vi "AB_850_860_Project_Source.vi"(7 "action":T4, 8 "error in (no error)":errorcluster, 9 "index in":i32, 10 "dataSource in":T3, 11 "buildObject":T1) -> (0 "error out":errorcluster, 1 "index out":i32, 2 "dataSource out":T3, 3 "buildObject out":T1)   [LabVIEW 2020]
doc: "Reads and writes the data to the object property bag."
uses:
  <resource>/Framework/Providers/API/ItemRef.ctl
  <vilib>/AppBuilder/AB_Source_Inclusion.ctl
  <vilib>/AppBuilder/RW_Project/AB_RW_Project_PropBag_Action.ctl
  <vilib>/AppBuilder/AB_Source_Property_WindowBehavior.ctl
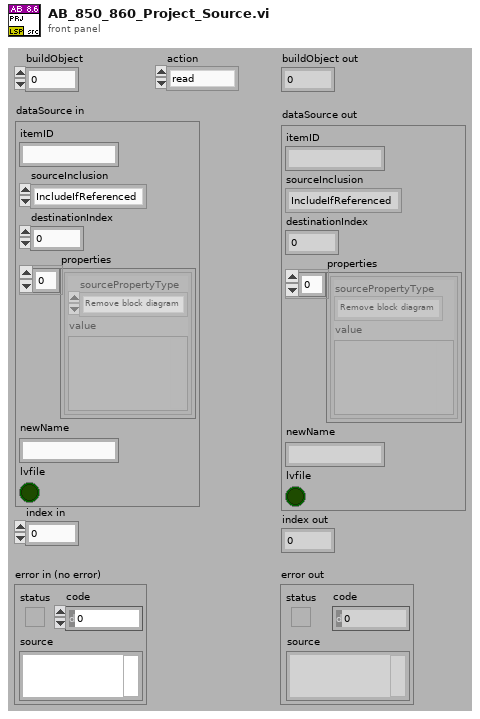
[diagram p1: front panel]
types:
  T1 = typedef "ItemRef.ctl" = u64
  T2 = typedef "AB_Source_Inclusion.ctl" = enum16{"IncludeIfReferenced", "Include", "Exclude", "TopLevel"}
  T3 = cluster{"itemID":string, "sourceInclusion":T2, "destinationIndex":i32, "properties":cluster{"sourcePropertyType":enum16{"Remove block diagram", "Remove front panel", "Password", "Window has title bar", "Show menu bar", "Show vertical scroll bar", "Show horizontal scroll bar", "Show toolbar", "Show Abort button", "Show fp when called", "Window behavior", "Allow user to close window", "Window run-time position", "Run when opened", "Allow debugging", "Auto error handling", "Generate guard code", "Use stack variables", "Expression folding", "Integer only", "Inline subVI"}, "value":variant}[], "newName":string, "lvfile":bool}
  T4 = typedef "AB_RW_Project_PropBag_Action.ctl" = enum16{"read", "write", "clear", "readPrevious", "writePrevious", "clearPrevious"}
  T5 = cluster{"sourcePropertyType":enum16{"Remove block diagram", "Remove front panel", "Password", "Window has title bar", "Show menu bar", "Show vertical scroll bar", "Show horizontal scroll bar", "Show toolbar", "Show Abort button", "Show fp when called", "Window behavior", "Allow user to close window", "Window run-time position", "Run when opened", "Allow debugging", "Auto error handling", "Generate guard code", "Use stack variables", "Expression folding", "Integer only", "Inline subVI"}, "value":variant}
  T6 = typedef "AB_Source_Property_WindowBehavior.ctl" = enum16{"Default", "Floating", "Modal"}
  T7 = enum16{"Remove block diagram", "Remove front panel", "Password", "Window has title bar", "Show menu bar", "Show vertical scroll bar", "Show horizontal scroll bar", "Show toolbar", "Show Abort button", "Show fp when called", "Window behavior", "Allow user to close window", "Window run-time position", "Run when opened", "Allow debugging", "Auto error handling", "Generate guard code", "Use stack variables", "Expression folding", "Integer only", "Inline subVI"}
  T8 = cluster{"sourcePropertyType":enum16{"Remove block diagram", "Remove front panel", "Password", "Window has title bar", "Show menu bar", "Show vertical scroll bar", "Show horizontal scroll bar", "Show toolbar", "Show Abort button", "Show fp when called", "Window behavior", "Allow user to close window", "Window run-time position", "Run when opened", "Allow debugging", "Auto error handling", "Generate guard code", "Use stack variables", "Expression folding", "Integer only", "Inline subVI"}, "value":variant}[]
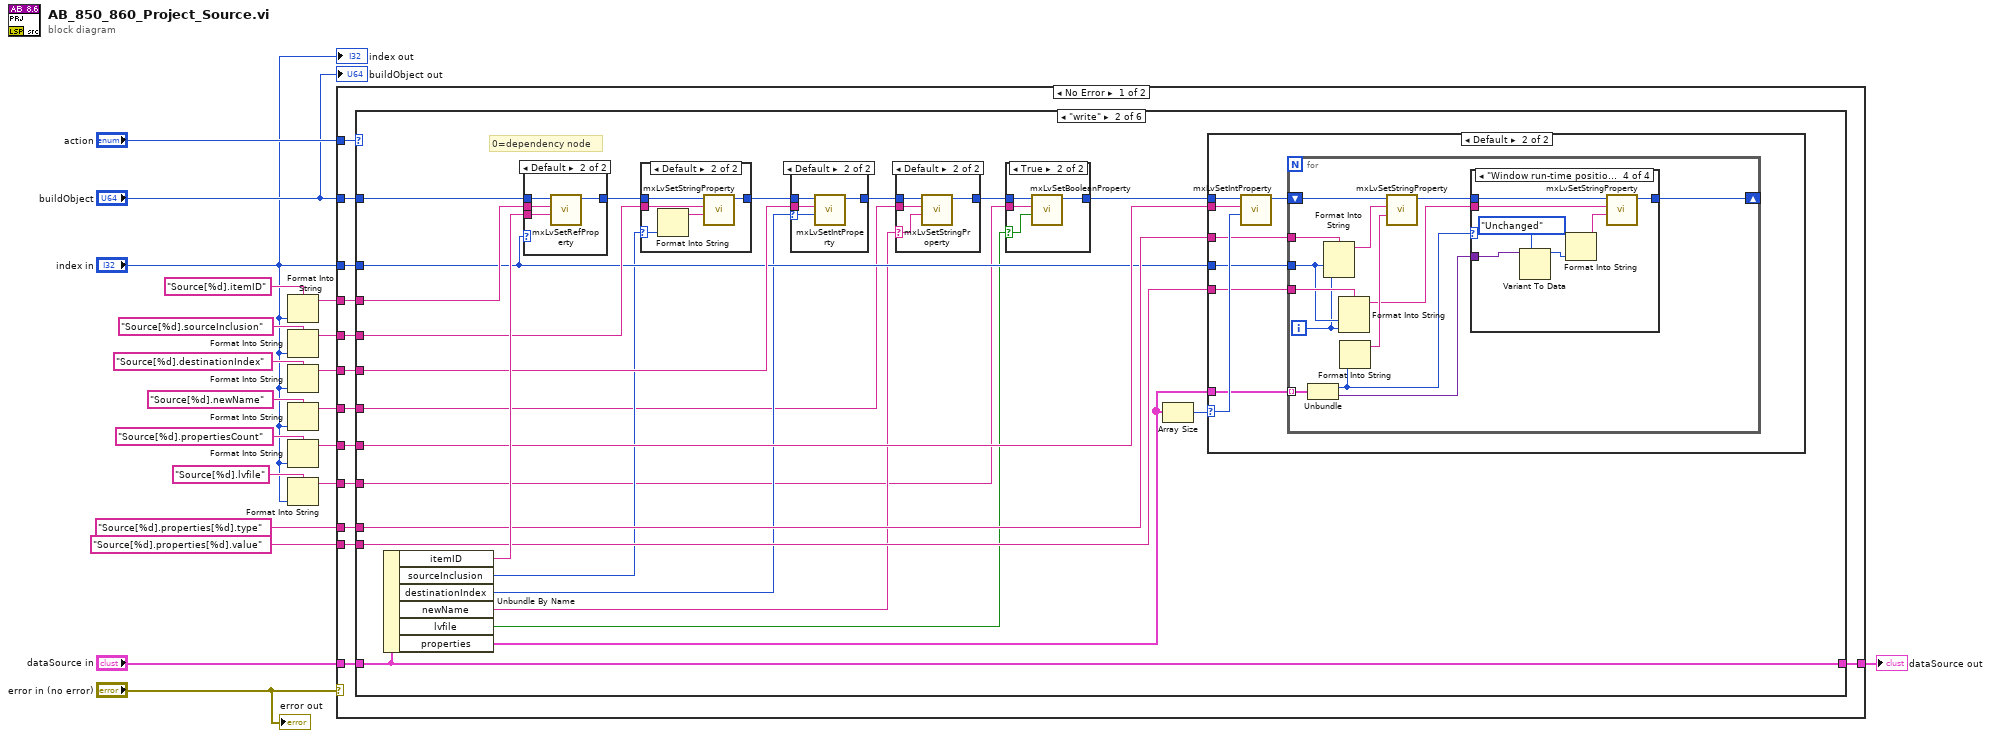
[diagram p0: block diagram]
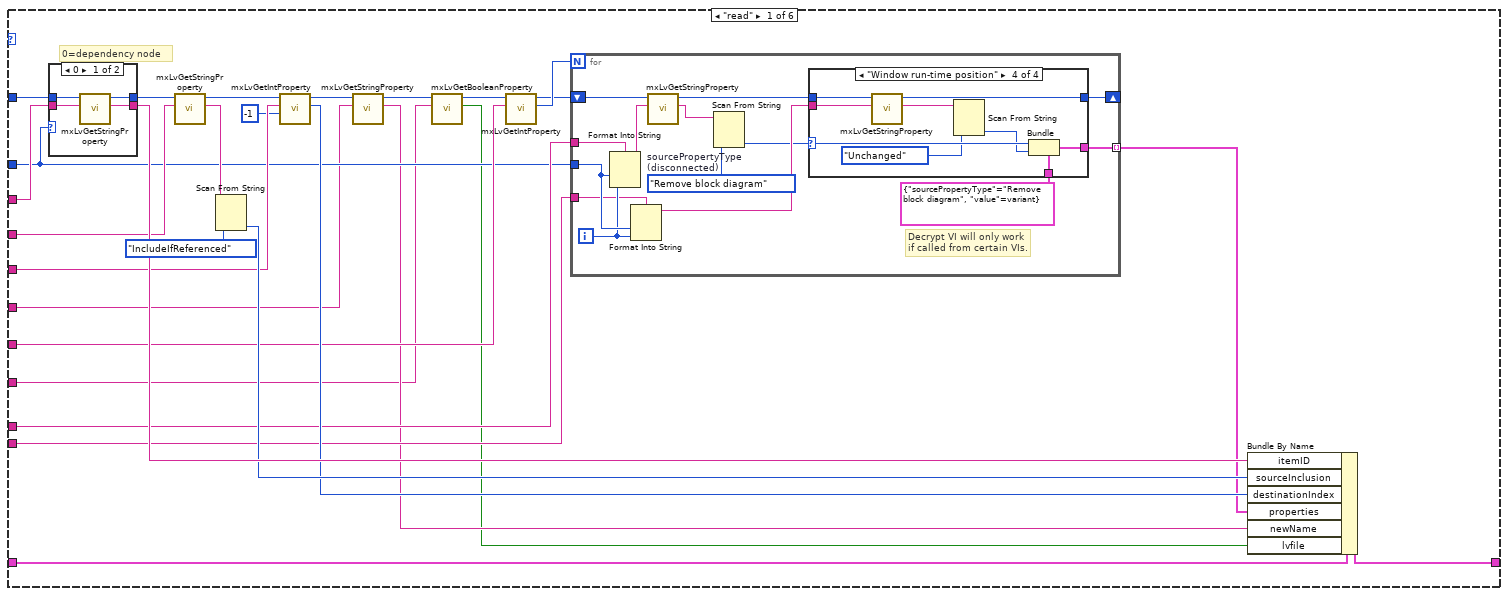
[diagram p2: hidden frame]
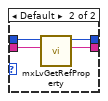
[diagram p3: hidden frame]
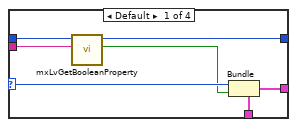
[diagram p4: hidden frame]
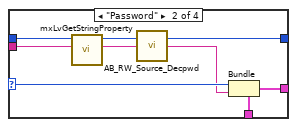
[diagram p5: hidden frame]
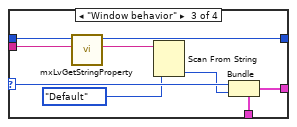
[diagram p6: hidden frame]
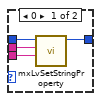
[diagram p11: hidden frame]
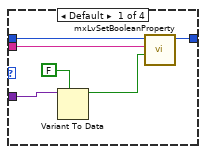
[diagram p13: hidden frame]
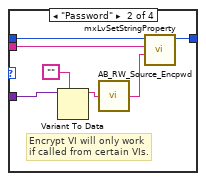
[diagram p14: hidden frame]
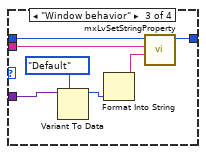
[diagram p15: hidden frame]
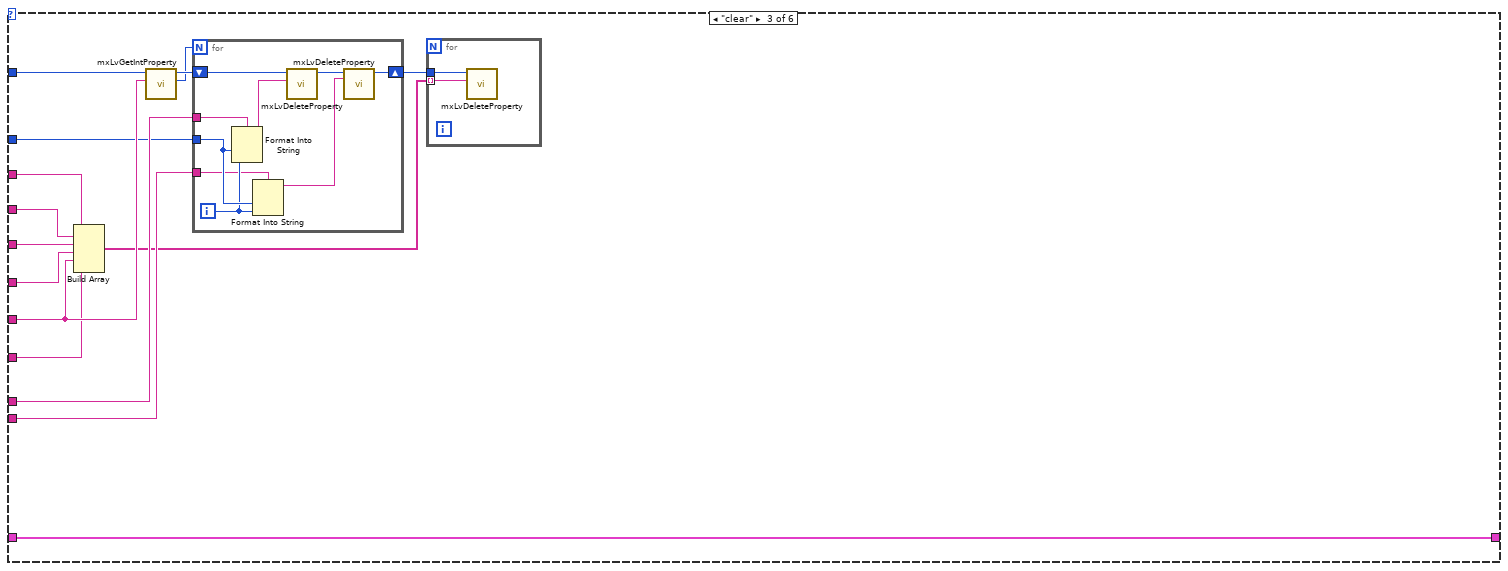
[diagram p16: hidden frame]
diagram:
  n1 = Format Into String(format string="Source[%d].itemID", "index in") -> (resulting string=w17:string)  [unwired: 2 in, 1 out]
  n2 = Format Into String(format string="Source[%d].sourceInclusion", "index in") -> (resulting string=w13:string)  [unwired: 2 in, 1 out]
  n3 = Format Into String(format string="Source[%d].destinationIndex", "index in") -> (resulting string=w12:string)  [unwired: 2 in, 1 out]
  n4 = Format Into String(format string="Source[%d].newName", "index in") -> (resulting string=w4:string)  [unwired: 2 in, 1 out]
  n5 = Format Into String(format string="Source[%d].propertiesCount", "index in") -> (resulting string=w11:string)  [unwired: 2 in, 1 out]
  n6 = Format Into String(format string="Source[%d].lvfile", "index in") -> (resulting string=w2:string)  [unwired: 2 in, 1 out]
  n7 = case shown="No Error" "error in (no error)" {
    tunnel: "action" -> [w33 _]
    tunnel: "dataSource in" -> [w32 w246]
    tunnel: w17 -> [w31 _]
    tunnel: w13 -> [w30 _]
    tunnel: w12 -> [w29 _]
    tunnel: w11 -> [w28 _]
    tunnel: "Source[%d].properties[%d].type" -> [w27 _]
    tunnel: "index in" -> [w26 _]
    tunnel: "Source[%d].properties[%d].value" -> [w25 _]
    tunnel: [w24 w246] -> w8
    tunnel: "buildObject" -> [w23 _]
    tunnel: w4 -> [w22 _]
    tunnel: w2 -> [w21 _]
    frame No Error {
      n8 = case shown="\"write\"" w33 {
        tunnel: w23 -> [w61 w138 w227 _ _ _]
        tunnel: w32 -> [w60 w139 w231 w243 w244 w245]
        tunnel: w31 -> [w58 w137 w230 _ _ _]
        tunnel: w30 -> [w56 w134 w229 _ _ _]
        tunnel: w29 -> [w51 w132 w228 _ _ _]
        tunnel: w28 -> [w49 w129 w225 _ _ _]
        tunnel: w27 -> [w47 w128 w223 _ _ _]
        tunnel: w26 -> [w42 w126 w221 _ _ _]
        tunnel: w25 -> [w45 w127 w222 _ _ _]
        tunnel: [w43 w139 w231 w243 w244 w245] -> w24
        tunnel: w22 -> [w39 w121 w218 _ _ _]
        tunnel: w21 -> [w37 w118 w217 _ _ _]
        frame "read" {
          # "0=dependency node"
          n9 = case shown="0" w42 {
            tunnel: w61 -> [w65 w69]
            tunnel: [w62 w68] -> w59
            tunnel: w58 -> [w63 w67]
            tunnel: [w64 w66] -> w57
            frame 0 {
              n10 = call <resource>:"mxLvGetStringProperty.vi"("Tag"=w63, "Item"=w65) -> ("Value"=w62:string, "Item"=w64:T1)  [unwired: 1 in, 7 out]
            }
            frame Default {
              n11 = call <resource>:"mxLvGetRefProperty.vi"("Tag"=w67, "Item"=w69) -> ("Value"=w68:string, "Item"=w66:T1)  [unwired: 1 in, 7 out]
            }
          }
          n12 = call <resource>:"mxLvGetStringProperty.vi"("Tag"=w56, "Item"=w57) -> ("Value"=w55:string, "Item"=w52:T1)  [unwired: 1 in, 7 out]
          n13 = Scan From String(input string=w55, default 1=AB_Source_Inclusion."IncludeIfReferenced" ("sourceInclusion")) -> (output 1=w53:T2)  [unwired: 3 in, 3 out]
          n14 = call <resource>:"mxLvGetIntProperty.vi"("Default Value (0)"=-1, "Tag"=w51, "Item"=w52) -> ("Value"=w50:i32, "Item"=w40:T1)  [unwired: 1 in, 6 out]
          n15 = call <resource>:"mxLvGetStringProperty.vi"("Tag"=w39, "Item"=w40) -> ("Value"=w38:string, "Item"=w35:T1)  [unwired: 1 in, 7 out]
          n16 = call <resource>:"mxLvGetBooleanProperty.vi"("Tag"=w37, "Item"=w35) -> ("Value"=w36:bool, "Item"=w34:T1)  [unwired: 1 in, 7 out]
          n17 = call <resource>:"mxLvGetIntProperty.vi"("Tag"=w49, "Item"=w34) -> ("Value"=w48:i32, "Item"=w46:T1)  [unwired: 1 in, 7 out]
          n18 = for {
            N: w48 -> [_]
            tunnel: w47 -> [w83]
            tunnel: w42 -> [w77]
            shift-right: [w73] -> _
            shift-left: w46 -> [w82]
            tunnel: w45 -> [w75]
            tunnel: [w71] -> w44 mode=indexing
            i -> [w76]
            w80 = T7."Remove block diagram"  # sourcePropertyType (disconnected)
            # "Decrypt VI will only work if called from certain VIs."
            n19 = Format Into String(format string=w83, w77, w76) -> (resulting string=w81:string)  [unwired: 2 in, 1 out]
            n20 = Format Into String(format string=w75, w77, w76) -> (resulting string=w74:string)  [unwired: 2 in, 1 out]
            n21 = call <resource>:"mxLvGetStringProperty.vi"("Tag"=w81, "Item"=w82) -> ("Value"=w79:string, "Item"=w78:T1)  [unwired: 1 in, 7 out]
            n22 = Scan From String(input string=w79, default 1=w80) -> (output 1=w72:T7)  [unwired: 3 in, 3 out]
            n23 = case shown="\"Window run-time position\"" w72 {
              selector: w72 -> [w87 w95 w104 w113]
              tunnel: w78 -> [w90 w98 w107 w116]
              tunnel: w74 -> [w89 w96 w105 w114]
              tunnel: [w88 w97 w106 w115] -> w73
              tunnel: [w85 w93 w102 w111] -> w71
              tunnel: T5 {"sourcePropertyType"=enum."Remove block diagram", "value"=variant} ("fileProperties") -> [w84 w94 w103 w112]
              frame Default {
                n24 = call <resource>:"mxLvGetBooleanProperty.vi"("Tag"=w89, "Item"=w90) -> ("Value"=w86:bool, "Item"=w88:T1)  [unwired: 1 in, 7 out]
                n25 = Bundle(cluster=w84, "sourcePropertyType"=w87, "value"=w86) -> (w85:T5)
              }
              frame "Password" {
                n26 = call <resource>:"mxLvGetStringProperty.vi"("Tag"=w96, "Item"=w98) -> ("Value"=w92:string, "Item"=w97:T1)  [unwired: 1 in, 7 out]
                n27 = call <vilib>:"AB_RW_Source_Decpwd.vi"("input string"=w92) -> ("output string"=w91:string)
                n28 = Bundle(cluster=w94, "sourcePropertyType"=w95, "value"=w91) -> (w93:T5)
              }
              frame "Window behavior" {
                n29 = call <resource>:"mxLvGetStringProperty.vi"("Tag"=w105, "Item"=w107) -> ("Value"=w101:string, "Item"=w106:T1)  [unwired: 1 in, 7 out]
                n30 = Scan From String(input string=w101, default 1=AB_Source_Property_WindowBehavior."Default" ("windowBehavior")) -> (output 1=w100:T6)  [unwired: 3 in, 3 out]
                n31 = Bundle(cluster=w103, "sourcePropertyType"=w104, "value"=w100) -> (w102:T5)
              }
              frame "Window run-time position" {
                n32 = call <resource>:"mxLvGetStringProperty.vi"("Tag"=w114, "Item"=w116) -> ("Value"=w110:string, "Item"=w115:T1)  [unwired: 1 in, 7 out]
                n33 = Scan From String(input string=w110, default 1=enum16{"Unchanged", "Centered", "Maximized"}."Unchanged" ("windowRunTimePosition")) -> (output 1=w109:enum16{"Unchanged", "Centered", "Maximized"})  [unwired: 3 in, 3 out]
                n34 = Bundle(cluster=w112, "sourcePropertyType"=w113, "value"=w109) -> (w111:T5)
              }
            }
          }
          n35 = Bundle By Name(cluster=w60, "itemID"=w59, "sourceInclusion"=w53, "destinationIndex"=w50, "properties"=w44, "newName"=w38, "lvfile"=w36) -> (w43:T3)
        }
        frame "write" {
          # "0=dependency node"
          n36 = Unbundle By Name(w139) -> ("itemID"=w136:string, "sourceInclusion"=w125:T2, "destinationIndex"=w124:i32, "newName"=w122:string, "lvfile"=w117:bool, "properties"=w131:T8)
          n37 = case shown="Default" w126 {
            tunnel: w138 -> [w164 w168]
            tunnel: w137 -> [w162 w167]
            tunnel: w136 -> [w161 w166]
            tunnel: [w163 w165] -> w135
            frame 0 {
              n38 = call <resource>:"mxLvSetStringProperty.vi"("Value (\"\")"=w161, "Tag"=w162, "Item"=w164) -> ("Item"=w163:T1)  [unwired: 2 in, 6 out]
            }
            frame Default {
              n39 = call <resource>:"mxLvSetRefProperty.vi"("Value (\"\")"=w166, "Tag"=w167, "Item"=w168) -> ("Item"=w165:T1)  [unwired: 2 in, 6 out]
            }
          }
          n40 = case shown="Default" w125 {
            selector: w125 -> [_ w156]
            tunnel: w135 -> [w155 w160]
            tunnel: w134 -> [_ w158]
            tunnel: [w155 w157] -> w133
            frame "IncludeIfReferenced" {
            }
            frame Default {
              n41 = Format Into String(w156) -> (resulting string=w159:string)  [unwired: 3 in, 1 out]
              n42 = call <resource>:"mxLvSetStringProperty.vi"("Value (\"\")"=w159, "Tag"=w158, "Item"=w160) -> ("Item"=w157:T1)  [unwired: 2 in, 6 out]
            }
          }
          n43 = case shown="Default" w124 {
            selector: w124 -> [_ w151]
            tunnel: w133 -> [w150 w154]
            tunnel: w132 -> [_ w153]
            tunnel: [w150 w152] -> w123
            frame -1 {
            }
            frame Default {
              n44 = call <resource>:"mxLvSetIntProperty.vi"("Value (0)"=w151, "Tag"=w153, "Item"=w154) -> ("Item"=w152:T1)  [unwired: 2 in, 6 out]
            }
          }
          n45 = case shown="Default" w122 {
            selector: w122 -> [_ w146]
            tunnel: w123 -> [w145 w149]
            tunnel: w121 -> [_ w148]
            tunnel: [w145 w147] -> w120
            frame "" {
            }
            frame Default {
              n46 = call <resource>:"mxLvSetStringProperty.vi"("Value (\"\")"=w146, "Tag"=w148, "Item"=w149) -> ("Item"=w147:T1)  [unwired: 2 in, 6 out]
            }
          }
          n47 = case shown="True" w117 {
            selector: w117 -> [_ w141]
            tunnel: w120 -> [w140 w144]
            tunnel: w118 -> [_ w143]
            tunnel: [w140 w142] -> w119
            frame False {
            }
            frame True {
              n48 = call <resource>:"mxLvSetBooleanProperty.vi"("Value (F)"=w141, "Tag"=w143, "Item"=w144) -> ("Item"=w142:T1)  [unwired: 2 in, 6 out]
            }
          }
          n49 = Array Size(array=w131) -> (size(s)=w130:i32)
          n50 = case shown="Default" w130 {
            selector: w130 -> [_ w174]
            tunnel: w131 -> [_ w172]
            tunnel: w129 -> [_ w176]
            tunnel: w119 -> [_ w175]
            tunnel: w128 -> [_ w171]
            tunnel: w126 -> [_ w170]
            tunnel: w127 -> [_ w169]
            frame 0 {
            }
            frame Default {
              n51 = call <resource>:"mxLvSetIntProperty.vi"("Value (0)"=w174, "Tag"=w176, "Item"=w175) -> ("Item"=w173:T1)  [unwired: 2 in, 6 out]
              n52 = for {
                shift-right: [w179] -> _
                shift-left: w173 -> [w189]
                tunnel: w172 -> [w188] mode=indexing
                tunnel: w171 -> [w187]
                tunnel: w170 -> [w183]
                tunnel: w169 -> [w184]
                i -> [w182]
                n53 = Unbundle(w188) -> ("sourcePropertyType"=w181:T7, "value"=w177:variant)
                n54 = Format Into String(format string=w187, w183, w182) -> (resulting string=w186:string)  [unwired: 2 in, 1 out]
                n55 = Format Into String(format string=w184, w183, w182) -> (resulting string=w178:string)  [unwired: 2 in, 1 out]
                n56 = Format Into String(w181) -> (resulting string=w185:string)  [unwired: 3 in, 1 out]
                n57 = call <resource>:"mxLvSetStringProperty.vi"("Value (\"\")"=w185, "Tag"=w186, "Item"=w189) -> ("Item"=w180:T1)  [unwired: 2 in, 6 out]
                n58 = case shown="\"Window run-time position\"" w181 {
                  tunnel: w180 -> [w195 w200 w208 w215]
                  tunnel: [w194 w199 w207 w214] -> w179
                  tunnel: w178 -> [w193 w198 w206 w213]
                  tunnel: w177 -> [w191 w202 w209 w216]
                  frame Default {
                    n59 = Variant To Data(type=FALSE, Variant=w191) -> (data=w190:bool)  [unwired: 1 in, 1 out]
                    n60 = call <resource>:"mxLvSetBooleanProperty.vi"("Value (F)"=w190, "Tag"=w193, "Item"=w195) -> ("Item"=w194:T1)  [unwired: 2 in, 6 out]
                  }
                  frame "Password" {
                    # "Encrypt VI will only work if called from certain VIs."
                    n61 = Variant To Data(type="", Variant=w202) -> (data=w197:string)  [unwired: 1 in, 1 out]
                    n62 = call <vilib>:"AB_RW_Source_Encpwd.vi"("input String"=w197) -> ("output String"=w196:string)  [unwired: 1 out]
                    n63 = call <resource>:"mxLvSetStringProperty.vi"("Value (\"\")"=w196, "Tag"=w198, "Item"=w200) -> ("Item"=w199:T1)  [unwired: 2 in, 6 out]
                  }
                  frame "Window behavior" {
                    n64 = Variant To Data(type=AB_Source_Property_WindowBehavior."Default" ("windowBehavior"), Variant=w209) -> (data=w204:T6)  [unwired: 1 in, 1 out]
                    n65 = Format Into String(w204) -> (resulting string=w203:string)  [unwired: 3 in, 1 out]
                    n66 = call <resource>:"mxLvSetStringProperty.vi"("Value (\"\")"=w203, "Tag"=w206, "Item"=w208) -> ("Item"=w207:T1)  [unwired: 2 in, 6 out]
                  }
                  frame "Window run-time position" {
                    n67 = Variant To Data(type=enum16{"Unchanged", "Centered", "Maximized"}."Unchanged" ("windowRunTimePosition"), Variant=w216) -> (data=w212:enum16{"Unchanged", "Centered", "Maximized"})  [unwired: 1 in, 1 out]
                    n68 = Format Into String(w212) -> (resulting string=w211:string)  [unwired: 3 in, 1 out]
                    n69 = call <resource>:"mxLvSetStringProperty.vi"("Value (\"\")"=w211, "Tag"=w213, "Item"=w215) -> ("Item"=w214:T1)  [unwired: 2 in, 6 out]
                  }
                }
              }
            }
          }
        }
        frame "clear" {
          n70 = Build Array(w230, w229, w228, w218, w225, w217) -> (w219:string[])
          n71 = call <resource>:"mxLvGetIntProperty.vi"("Tag"=w225, "Item"=w227) -> ("Value"=w224:i32, "Item"=w226:T1)  [unwired: 1 in, 7 out]
          n72 = for {
            N: w224 -> [_]
            tunnel: w223 -> [w242]
            tunnel: w221 -> [w241]
            shift-right: [w236] -> w220
            shift-left: w226 -> [w238]
            tunnel: w222 -> [w239]
            i -> [w240]
            n73 = Format Into String(format string=w242, w241, w240) -> (resulting string=w235:string)  [unwired: 2 in, 1 out]
            n74 = Format Into String(format string=w239, w241, w240) -> (resulting string=w234:string)  [unwired: 2 in, 1 out]
            n75 = call <resource>:"mxLvDeleteProperty.vi"("Tag"=w235, "Item"=w238) -> ("Item"=w237:T1)  [unwired: 1 in, 8 out]
            n76 = call <resource>:"mxLvDeleteProperty.vi"("Tag"=w234, "Item"=w237) -> ("Item"=w236:T1)  [unwired: 1 in, 8 out]
          }
          n77 = for {
            tunnel: w220 -> [w233]
            tunnel: w219 -> [w232] mode=indexing
            n78 = call <resource>:"mxLvDeleteProperty.vi"("Tag"=w232, "Item"=w233) -> ()  [unwired: 1 in, 9 out]
          }
        }
        frame "readPrevious" {
        }
        frame "writePrevious" {
        }
        frame "clearPrevious" {
        }
      }
    }
    frame Error {
    }
  }
  "dataSource out" <- w8
  "error out" <- "error in (no error)"
  "buildObject out" <- "buildObject"
  "index out" <- "index in"
